vi "清楚数组空元素.vi"(5 "Value":string[](array[string])) -> (2 "已删除元素的数组子集":string[](array[string]))   [LabVIEW 2016, in "数据传输系统.lvlib" / "自动更新.lvlib" / "TCP文件传输系统.lvlib" / "TCP接收文件.lvlib"]
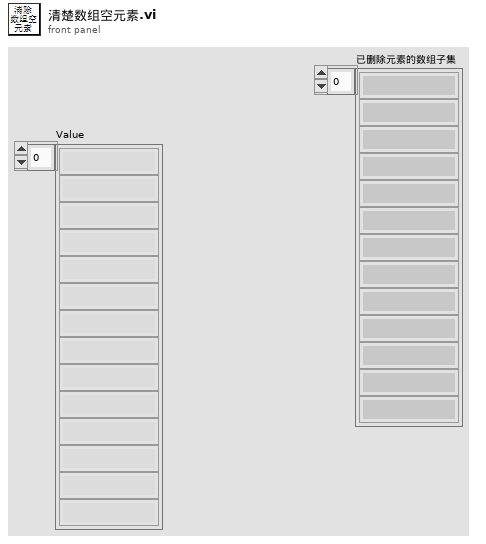
[diagram p1: front panel]
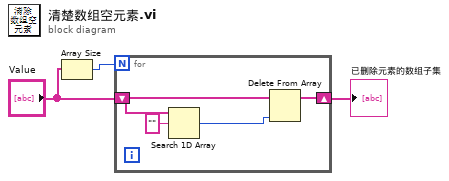
[diagram p0: block diagram]
diagram:
  n1 = Array Size(array="Value") -> (size(s)=w1:i32)
  n2 = for {
    N: w1 -> [_]
    shift-right: [w4] -> w3
    shift-left: "Value" -> [w6]
    n3 = Search 1D Array(1D array=w6, element="" ("元素")) -> (index of element=w5:i32)  [unwired: 1 in]
    n4 = Delete From Array(array=w6, index=w5) -> (array with subset deleted=w4:string[])  [unwired: 1 in, 1 out]
  }
  "已删除元素的数组子集" <- w3
